vi "Test App Broadcast Owned Process Messages.vi"(8 "error in (no error)":errorcluster, 11 "Application Test In":refnum<class "Application Dev Test.lvclass">) -> (0 "error out":errorcluster, 3 "Application Test Out":refnum<class "Application Dev Test.lvclass">)   [LabVIEW 2020, in "Application Dev Test.lvclass"]
uses:
  Application Dev Test.lvclass
  C:/Program Files (x86)/National Instruments/LabVIEW 2020/vi.lib/Astemes/LUnit/Test Case.lvclass
  source/Framework Test Suite/Mock Process/Mock Process.lvclass
  C:/git/astemes-triarc-framework/source/Framework/Process/Process.lvclass
  source/Framework/Process/Process.lvclass/Process.ctl
  <vilib>/Astemes/LUnit/Test Case.lvclass/Test Case.ctl
  d7aac43e-207c-41c6-a8df-6345f13d1659.vi
  17ad9605-3f1d-49a9-a18e-9fbc0b2c3033.vi
  fa850677-95b7-4037-93e7-476298c3a011.vi
  source/Framework/Process/Private/SubVIs/Wait for finish.vi
  source/Framework/Process/Private/SubVIs/Set Lifecycle State.vi
  source/Framework/Process/Protected/Messaging/Send Message.vi
  <vilib>/Astemes/LUnit/Append Pass Result.vi
  <vilib>/Astemes/LUnit/Append Fail Result.vi
  d7aac43e-207c-41c6-a8df-6345f13d1659.vi/9c5d11cd-9439-4240-a1ee-d9baace9c924.vi
  17ad9605-3f1d-49a9-a18e-9fbc0b2c3033.vi/9c5d11cd-9439-4240-a1ee-d9baace9c924.vi
  fa850677-95b7-4037-93e7-476298c3a011.vi/9c5d11cd-9439-4240-a1ee-d9baace9c924.vi
  source/Framework/Process/Private/SubVIs/Handle Debug Data.vi
  <vilib>/Astemes/LUnit/Run In UI.vi
  source/Framework/Logging/Log Debug.vi
  <vilib>/AdvancedString/1D String Array to Delimited String.vi
  <vilib>/Utility/High Resolution Relative Seconds.vi
  <vilib>/Utility/error.llb/Clear Errors.vi
  source/Framework/Application/Application.lvclass
  source/Framework/Process/Public/Lifecycle/Get Lifecycle State.vi
  <vilib>/Utility/error.llb/Error Cluster From Error Code.vi
  source/Framework/Process/Public/Read Name.vi
  source/Framework/Callback/Callback.lvclass
  source/Framework/Process/Process.lvclass
  source/Framework/Broadcast Event Dequeuers/Broadcast Event Dequeuers.lvlib
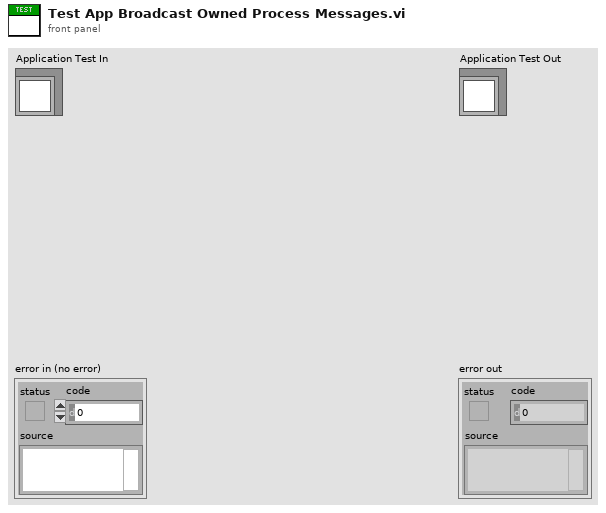
[diagram p1: front panel]
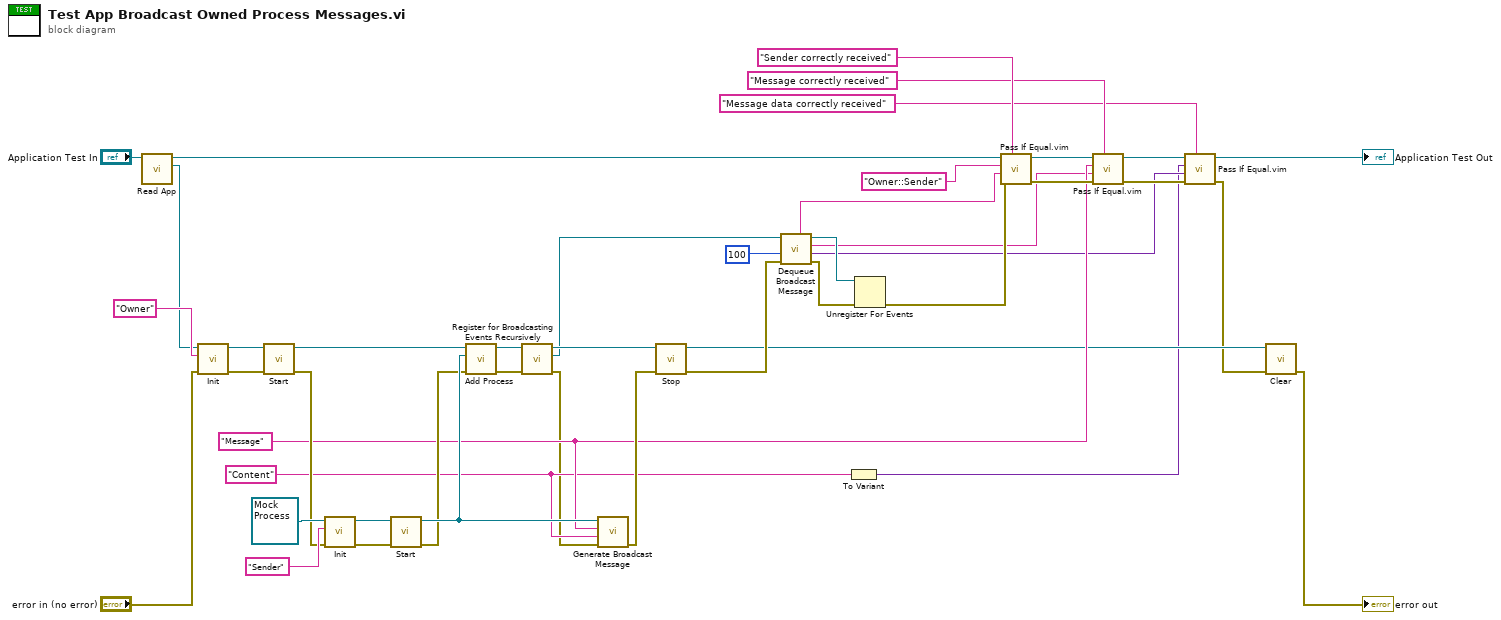
[diagram p0: block diagram]
diagram:
  w14 = "Content" ("Message")
  w15 = "Message" ("Message")
  n1 = call "Read App.vi"("Application Test In"="Application Test In") -> ("App out"=w22:refnum<class "Application.lvclass">, "Application Test Out"=w23:refnum<class "Application Dev Test.lvclass">)  [unwired: 8 in, 1 out]
  n2 = call-dynamic "Init.vi"("error in (no error)"="error in (no error)", "Name"="Owner" ("Message"), "Process In"=w22) -> ("error out"=w43:errorcluster, "Process Out"=w44:refnum<class "Application.lvclass">)  [unwired: 7 in]
  n3 = call "Start.vi"("error in (no error)"=w43, "Process In"=w44) -> ("error out"=w17:errorcluster, "Process Out"=w40:refnum<class "Application.lvclass">)  [unwired: 7 in, 1 out]
  n4 = call-dynamic "Init.vi"("error in (no error)"=w17, "Name"="Sender" ("Message"), "Mock Process In"=refnum<class "Mock Process.lvclass"> refnum ("Mock Process.lvclass")) -> ("error out"=w26:errorcluster, "Mock Process Out"=w25:refnum<class "Mock Process.lvclass">)  [unwired: 7 in]
  n5 = call "Start.vi"("error in (no error)"=w26, "Process In"=w25) -> ("error out"=w16:errorcluster, "Process Out"=w21:refnum<class "Mock Process.lvclass">)  [unwired: 7 in, 1 out]
  n6 = call "Add Process.vi"("error in (no error)"=w16, "Process"=w21, "Application In"=w40) -> ("error out"=w8:errorcluster, "Application Out"=w9:refnum<class "Application.lvclass">)  [unwired: 7 in]
  n7 = call "Register for Broadcasting Events Recursively.vi"("error in (no error)"=w8, "Application In"=w9) -> ("error out"=w6:errorcluster, "Event Registration Refnum Out"=w5:refnum<event-registration>, "Application Out"=w7:refnum<class "Application.lvclass">)  [unwired: 7 in]
  n8 = call "Generate Broadcast Message.vi"("error in (no error)"=w6, "Message Data"=w14, "Message"=w15, "Mock Process In"=w21) -> ("error out"=w19:errorcluster)  [unwired: 6 in, 1 out]
  n9 = call "Stop.vi"("error in (no error)"=w19, "Process In"=w7) -> ("error out"=w42:errorcluster, "Process Out"=w4:refnum<class "Application.lvclass">)  [unwired: 7 in, 1 out]
  n10 = call "Dequeue Broadcast Message.vi"("error in (no error)"=w42, "Timeout (-1)"=100, "Event Registration Refnum"=w5) -> ("error out"=w10:errorcluster, "Message Data"=w12:variant, "Message"=w13:string, "Event Registration Refnum Out"=w39:refnum<event-registration>, "Sender"=w38:string)  [unwired: 3 in, 1 out]
  n11 = To Variant(anything=w14) -> (Variant=w1:variant)
  n12 = Unregister For Events(event registration refnum=w39, error in=w10) -> (error out=w32:errorcluster)
  n13 = call "Pass If Equal.vim"("Description"="Sender correctly received", "error in (no error)"=w32, "Actual"=w38, "Expected"="Owner::Sender" ("Message"), "LUnit Test Case In"=w23) -> ("error out"=w35:errorcluster, "LUnit Test Case Out"=w36:refnum<class "Application Dev Test.lvclass">)  [unwired: 5 in]
  n14 = call "Pass If Equal.vim"("Description"="Message correctly received", "error in (no error)"=w35, "Actual"=w13, "Expected"=w15, "LUnit Test Case In"=w36) -> ("error out"=w33:errorcluster, "LUnit Test Case Out"=w34:refnum<class "Application Dev Test.lvclass">)  [unwired: 5 in]
  n15 = call "Pass If Equal.vim"("Description"="Message data correctly received", "error in (no error)"=w33, "Actual"=w12, "Expected"=w1, "LUnit Test Case In"=w34) -> ("error out"=w3:errorcluster, "LUnit Test Case Out"=→"Application Test Out":refnum<class "Application Dev Test.lvclass">)  [unwired: 5 in]
  n16 = call-dynamic "Clear.vi"("error in (no error)"=w3, "Application In"=w4) -> ("error out"=→"error out":errorcluster)  [unwired: 9 in]
